vi "Command_Position.vi"() -> ()   [LabVIEW 2018]
panel:
  out "Command_Position":dbl[](array[numeric])
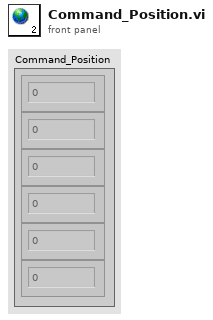
[diagram p1: front panel]
diagram:
